vi "get software root directory.vi"() -> (3 "Application Directory":path)   [LabVIEW 2013]
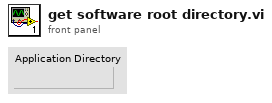
[diagram p1: front panel]
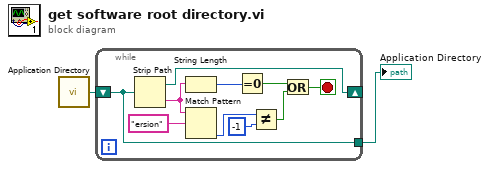
[diagram p0: block diagram]
diagram:
  n1 = call <vilib>:"Application Directory.vi"() -> ("Application Directory"=w1:path)
  n2 = while {
    shift-right: [w12] -> _
    shift-left: w1 -> [w3]
    tunnel: [w3] -> w2
    stop <- w4 stop-if-true
    n3 = Strip Path(path=w3) -> (stripped path=w12:path, name=w7:string)
    n4 = String Length(string=w7) -> (length=w6:i32)
    n5 = Match Pattern(string=w7, regular expression="ersion") -> (offset past match=w11:i32)  [unwired: 1 in, 3 out]
    n6 = Equal To 0?(x=w6) -> (x = 0?=w5:bool)
    n7 = Not Equal?(x=w11, y=-1) -> (x != y?=w8:bool)
    n8 = Or(x=w5, y=w8) -> (x .or. y?=w4:bool)
  }
  "Application Directory" <- w2
